vi "Multiply_4channel.vi"(8 "DDS Sine":fxp<+/-,16,0>[](array[numeric])=[0.0, 0.0, 0.0, 0.0], 9 "DDS Cosine":fxp<+/-,16,0>[](array[numeric])=[0.0, 0.0, 0.0, 0.0], 11 "Signal Input":i16[](array[numeric])=[0, 0, 0, 0]) -> (1 "Q output":fxp<+/-,16,14>[](array[numeric]), 2 "I output":fxp<+/-,16,14>[](array[numeric]))   [LabVIEW 2013]
doc: "I-Q Multiplyer for 4Ch input. (Frequency transfer.)\nOutput: FXP: +- 16,14"
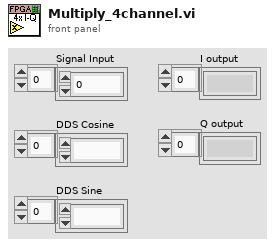
[diagram p1: front panel]
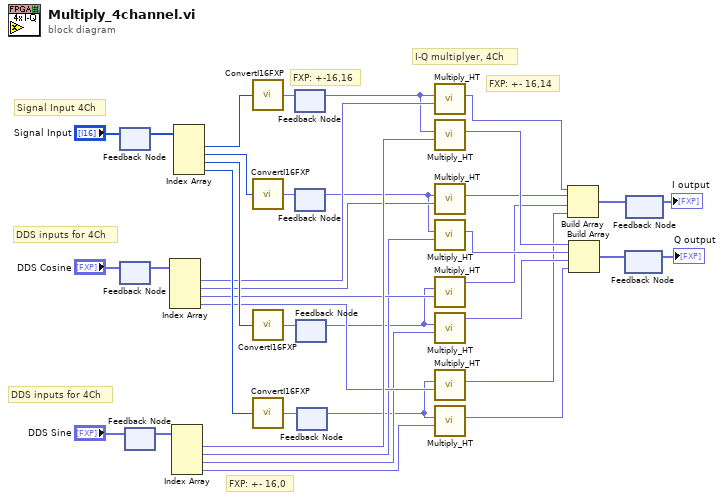
[diagram p0: block diagram]
diagram:
  # "FXP: +- 16,14"
  # "FXP: +- 16,0"
  # "FXP: +-16,16"
  # "DDS inputs for 4Ch"
  # "DDS inputs for 4Ch"
  # "Signal Input 4Ch"
  # "I-Q multiplyer, 4Ch"
  n1 = feedback-in #1("Signal Input") -> ()
  n2 = feedback #1() -> (w9:i16[])  [unwired: 1 in]
  n3 = feedback #2() -> (w7:fxp<+/-,16,0>[])  [unwired: 1 in]
  n4 = feedback-in #2("DDS Cosine") -> ()
  n5 = feedback #3() -> (w5:fxp<+/-,16,0>[])  [unwired: 1 in]
  n6 = feedback-in #3("DDS Sine") -> ()
  n7 = Index Array(array=w7) -> (element #1=w34:fxp<+/-,16,0>, element #2=w32:fxp<+/-,16,0>, element #3=w31:fxp<+/-,16,0>, element #4=w30:fxp<+/-,16,0>)  [unwired: 4 in]
  n8 = Index Array(array=w5) -> (element #1=w33:fxp<+/-,16,0>, element #2=w29:fxp<+/-,16,0>, element #3=w28:fxp<+/-,16,0>, element #4=w27:fxp<+/-,16,0>)  [unwired: 4 in]
  n9 = Index Array(array=w9) -> (element #1=w35:i16, element #2=w36:i16, element #3=w37:i16, element #4=w38:i16)  [unwired: 4 in]
  n10 = call "ConvertI16FXP.vi"("I16"=w35) -> ("y"=w26:fxp<+/-,16,16>)
  n11 = call "ConvertI16FXP.vi"("I16"=w36) -> ("y"=w24:fxp<+/-,16,16>)
  n12 = call "ConvertI16FXP.vi"("I16"=w37) -> ("y"=w22:fxp<+/-,16,16>)
  n13 = call "ConvertI16FXP.vi"("I16"=w38) -> ("y"=w20:fxp<+/-,16,16>)
  n14 = feedback #4() -> (w25:fxp<+/-,16,16>)  [unwired: 1 in]
  n15 = feedback-in #4(w26) -> ()
  n16 = feedback #5() -> (w23:fxp<+/-,16,16>)  [unwired: 1 in]
  n17 = feedback-in #5(w24) -> ()
  n18 = feedback #6() -> (w21:fxp<+/-,16,16>)  [unwired: 1 in]
  n19 = feedback-in #6(w22) -> ()
  n20 = feedback #7() -> (w19:fxp<+/-,16,16>)  [unwired: 1 in]
  n21 = feedback-in #7(w20) -> ()
  n22 = call "Multiply_HT.vi"("DDS sample"=w34, "Signal sample"=w25) -> ("Output"=w18:fxp<+/-,16,14>)  [unwired: 8 in, 1 out]
  n23 = call "Multiply_HT.vi"("DDS sample"=w33, "Signal sample"=w25) -> ("Output"=w17:fxp<+/-,16,14>)  [unwired: 8 in, 1 out]
  n24 = call "Multiply_HT.vi"("DDS sample"=w32, "Signal sample"=w23) -> ("Output"=w16:fxp<+/-,16,14>)  [unwired: 8 in, 1 out]
  n25 = call "Multiply_HT.vi"("DDS sample"=w29, "Signal sample"=w23) -> ("Output"=w15:fxp<+/-,16,14>)  [unwired: 8 in, 1 out]
  n26 = call "Multiply_HT.vi"("DDS sample"=w31, "Signal sample"=w21) -> ("Output"=w14:fxp<+/-,16,14>)  [unwired: 8 in, 1 out]
  n27 = call "Multiply_HT.vi"("DDS sample"=w28, "Signal sample"=w21) -> ("Output"=w13:fxp<+/-,16,14>)  [unwired: 8 in, 1 out]
  n28 = call "Multiply_HT.vi"("DDS sample"=w30, "Signal sample"=w19) -> ("Output"=w12:fxp<+/-,16,14>)  [unwired: 8 in, 1 out]
  n29 = call "Multiply_HT.vi"("DDS sample"=w27, "Signal sample"=w19) -> ("Output"=w11:fxp<+/-,16,14>)  [unwired: 8 in, 1 out]
  n30 = Build Array(w18, w16, w14, w12) -> (w4:fxp<+/-,16,14>[])
  n31 = Build Array(w17, w15, w13, w11) -> (w2:fxp<+/-,16,14>[])
  n32 = feedback #8() -> (→"Q output":fxp<+/-,16,14>[])  [unwired: 1 in]
  n33 = feedback-in #8(w2) -> ()
  n34 = feedback #9() -> (→"I output":fxp<+/-,16,14>[])  [unwired: 1 in]
  n35 = feedback-in #9(w4) -> ()
